vi "2. CoffeeMaker State Machine.vi"() -> ()   [LabVIEW 2018]
doc: "Coffee Machine Version 1.0: using a state machine as program structure"
uses:
  Controls/States.ctl
panel:
  out "error out":errorcluster
  in  "error in (no error)":errorcluster
  in  "Power Switch":bool
  in  "Simulation":cluster{"Water":dbl, "Coffee":dbl, "Milk":dbl} {"Milk" scale=0.0..100.0; "Water" scale=0.0..100.0; "Coffee" scale=0.0..100.0}
  out "Display":T1 {"Coffee" scale=0.0..80.0; "Brewing Chamber" scale=0.0..80.0}
  in  "Control Elements":T2 {"Type" min=0 max=2 scale=0.0..2.0}
  # "Coffee Selection"
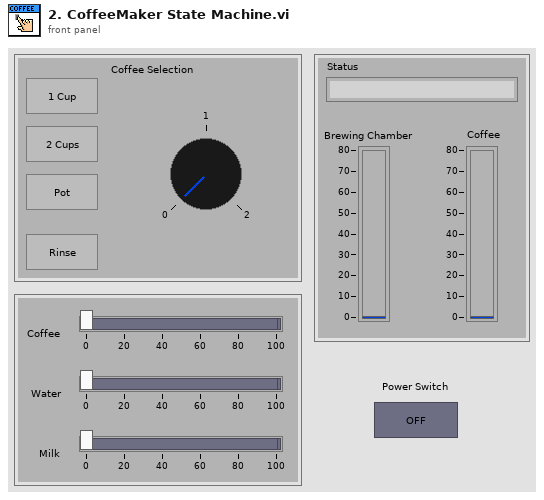
[diagram p1: front panel]
types:
  T1 = cluster{"Brewing Chamber":dbl, "Coffee":dbl, "Status":string}
  T2 = cluster{"1 Cup":bool, "2 Cups":bool, "Pot":bool, "Rinse":bool, "Type":i8}
  T3 = typedef "States.ctl" = enum16{"Initialize", "Set Language", "Wait for Power On", "Heat up", "Check and Wait for Water", "Rinsing", "Check Resources", "User Input", "Grinding", "Boiling", "Pouring", "Rinse before Stop", "Write Data", "Stop"}
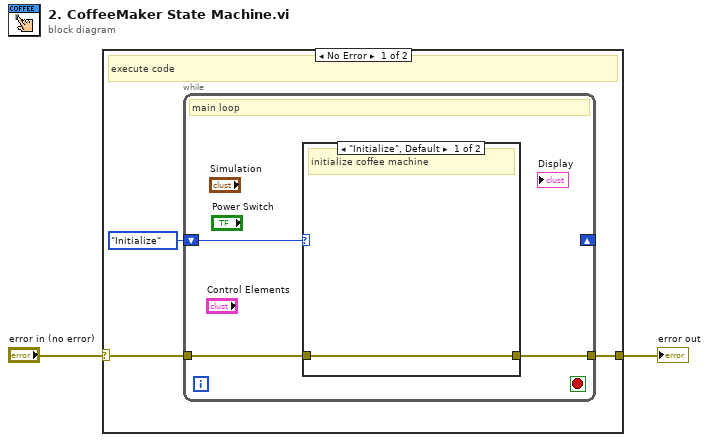
[diagram p0: block diagram]
diagram:
  n1 = case shown="No Error" "error in (no error)" {
    selector: "error in (no error)" -> [w4 w11]
    tunnel: [w5 w11] -> w1
    frame No Error {
      # "execute code"
      n2 = while {
        tunnel: [w7] -> w5
        tunnel: w4 -> [w6]
        shift-right: _ -> [_]
        shift-left: States."Initialize" -> [w8]
        stop <- _ stop-if-true
        # "main loop"
        n3 = case shown="\"Initialize\", Default" w8 {
          tunnel: [w9 w10] -> w7
          tunnel: w6 -> [w9 w10]
          frame "Initialize", Default {
            # "initialize coffee machine"
          }
          frame "Set Language" {
          }
        }
      }
    }
    frame Error {
      # "do nothing"
    }
  }
  "error out" <- w1
